vi "JKI.vi"() -> ()   [LabVIEW 2020]
uses:
  <userlib>/sushu/Tools/Front Panel State.ctl
  <vilib>/Utility/error.llb/Trim Whitespace.vi
  <userlib>/sushu/sushu.lvlib
panel:
  in  "OK":bool
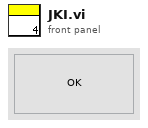
[diagram p1: front panel]
types:
  T1 = cluster{"Current VI Reference":refnum<vi>, "Close Panel on Exit?":bool}
  T2 = cluster{"Core":cluster{"Current VI Reference":refnum<vi>, "Close Panel on Exit?":bool}}
  T3 = enum32{"invalid app kind", "Development System", "Run Time System", "Student Edition", "Embedded LabVIEW", "Evaluation", "Custom"}
  T4 = typedef "sushu.lvlib/Front Panel State.ctl" = string
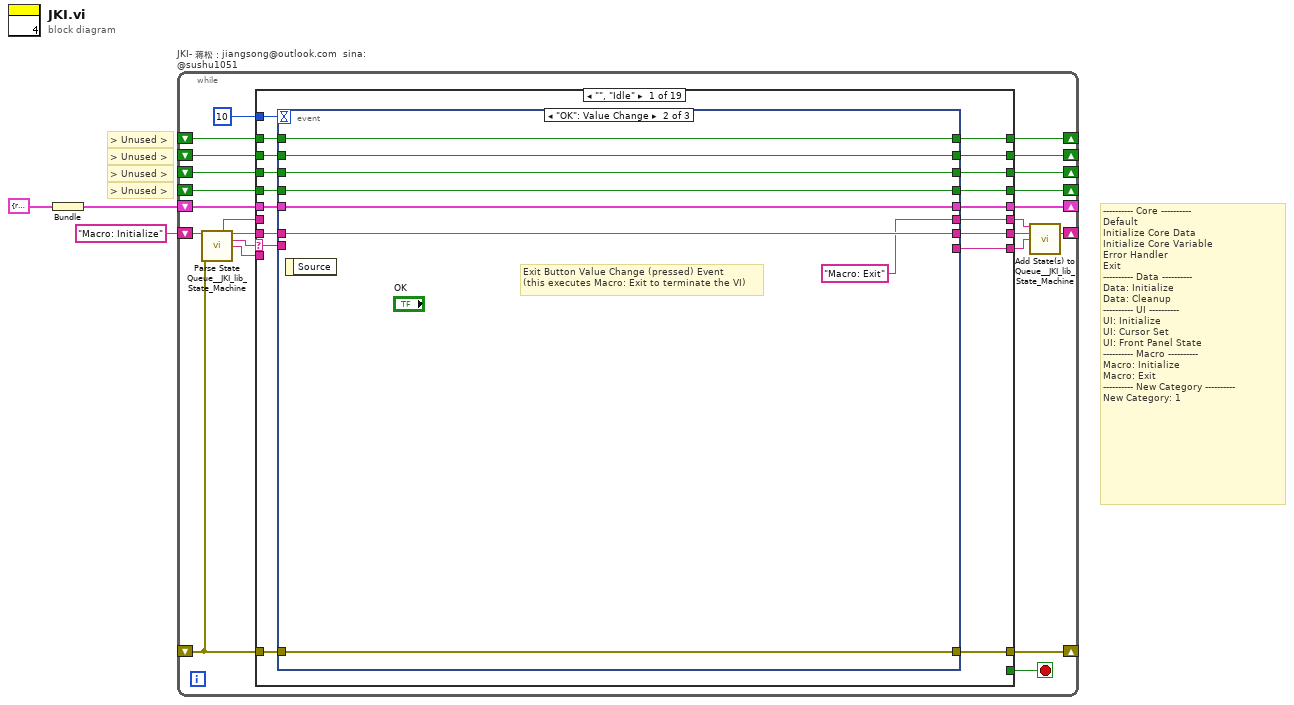
[diagram p0: block diagram]
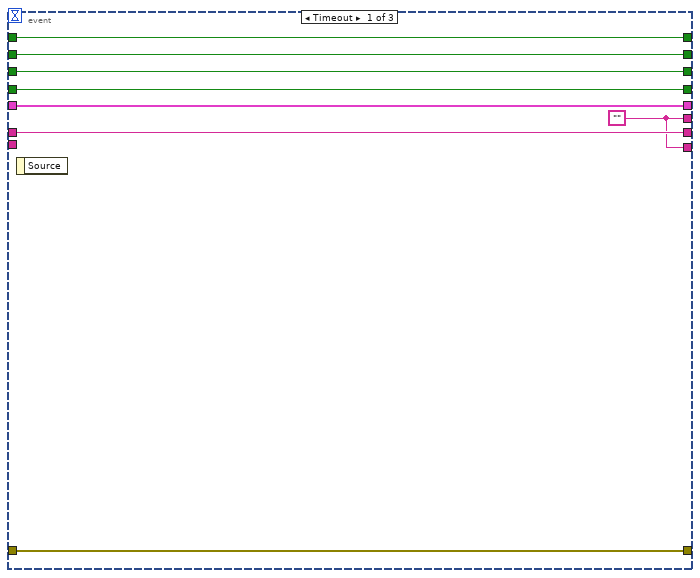
[diagram p2: hidden frame]
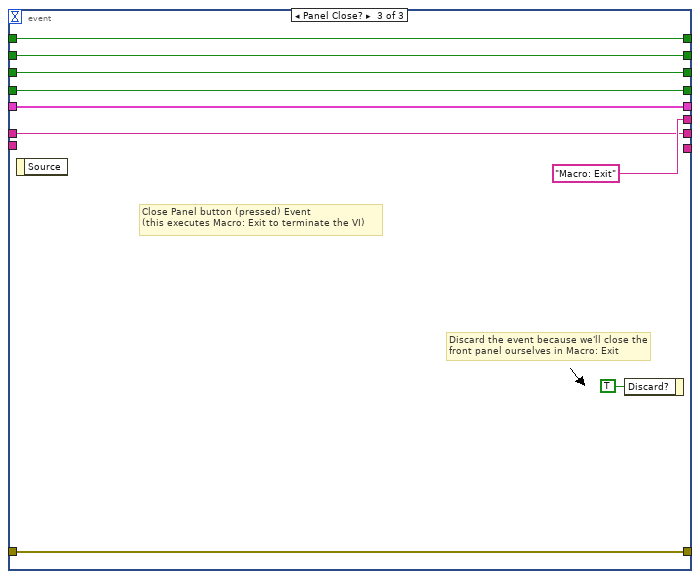
[diagram p3: hidden frame]
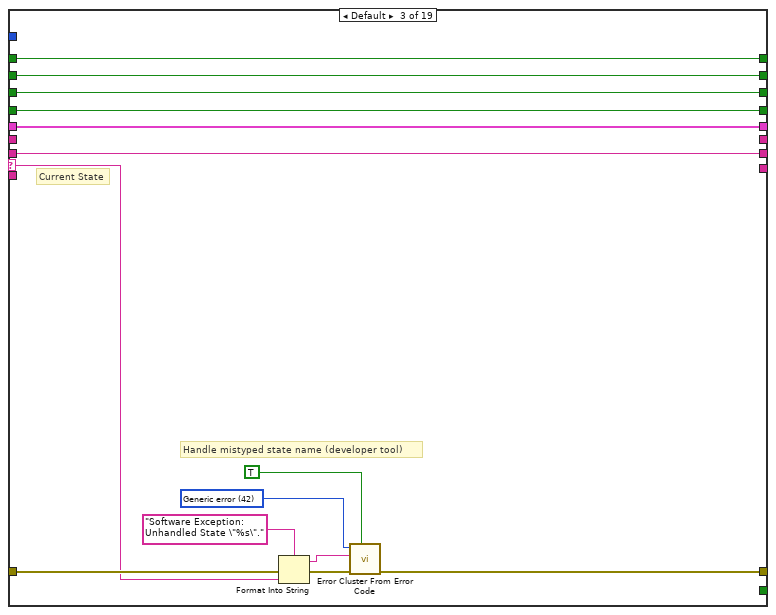
[diagram p5: hidden frame]
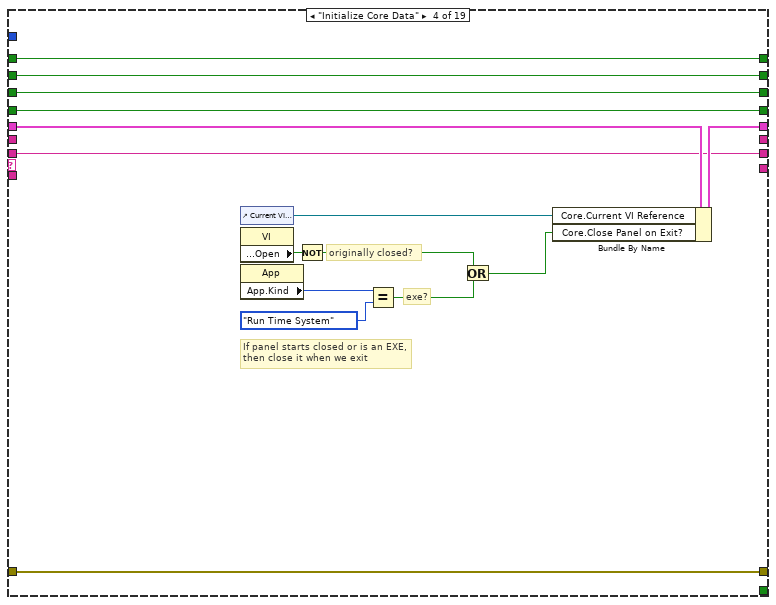
[diagram p6: hidden frame]
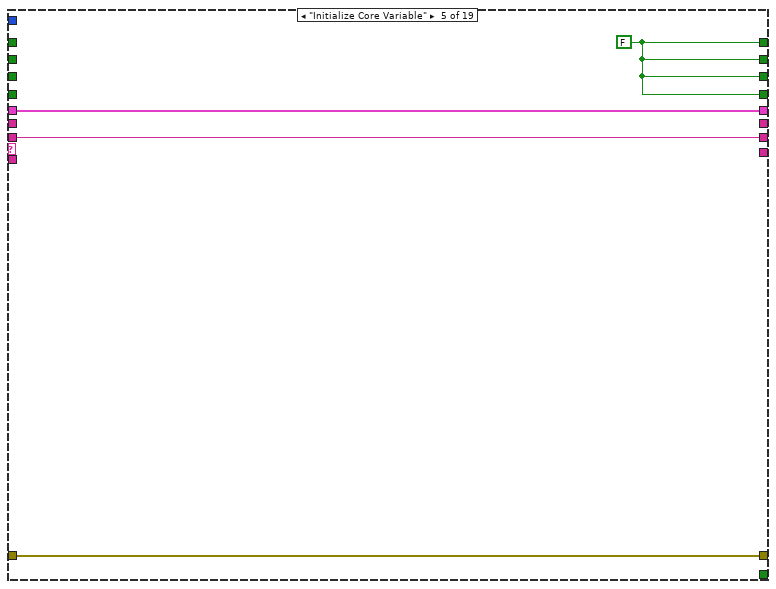
[diagram p7: hidden frame]
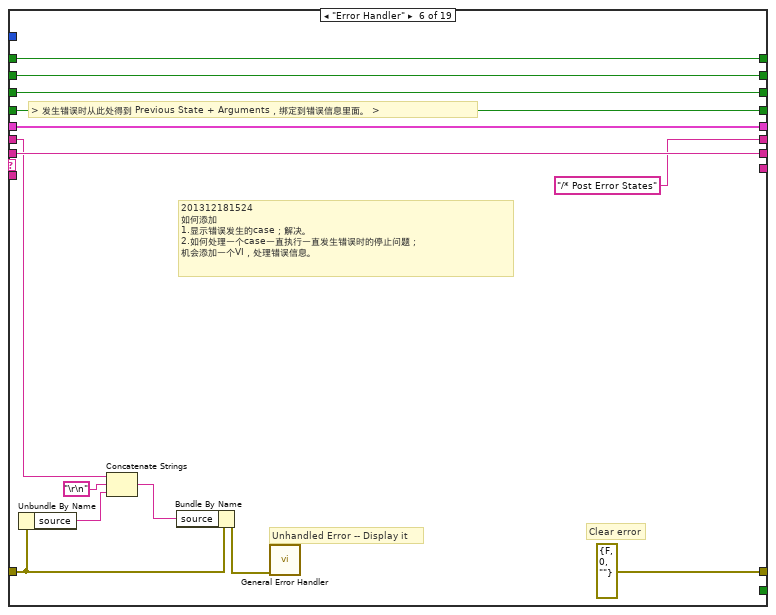
[diagram p8: hidden frame]
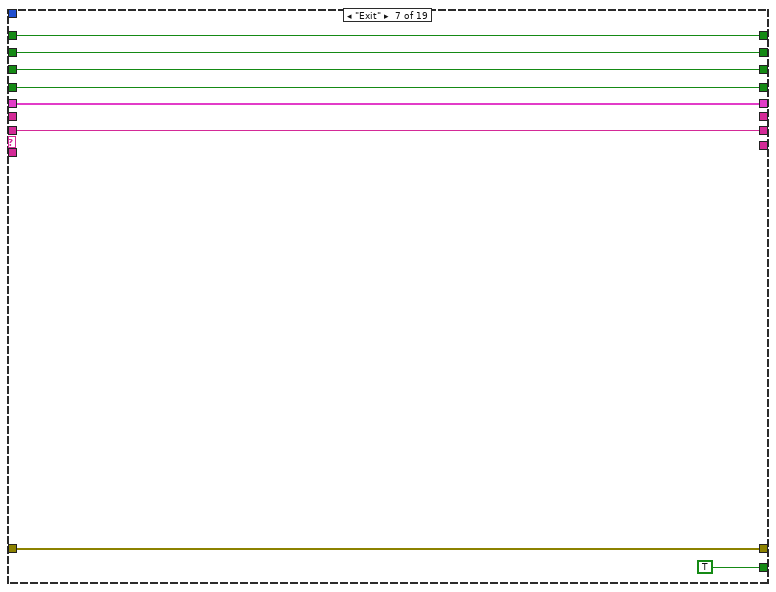
[diagram p9: hidden frame]
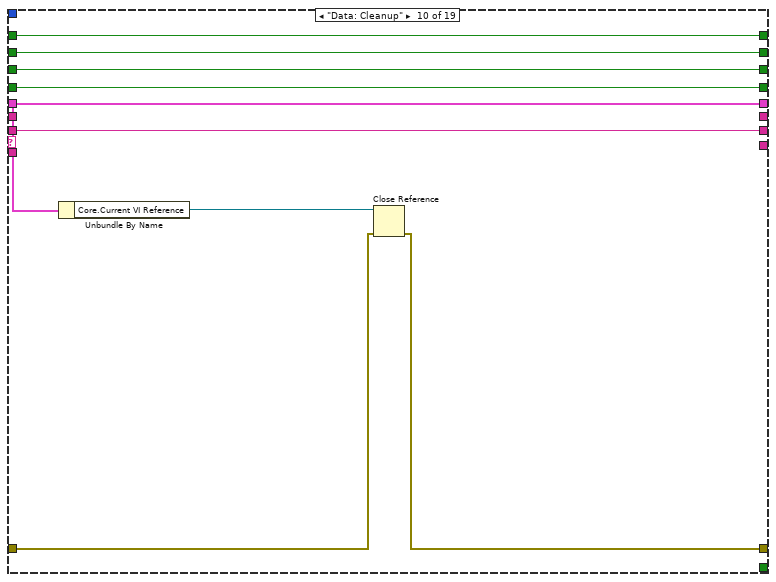
[diagram p12: hidden frame]
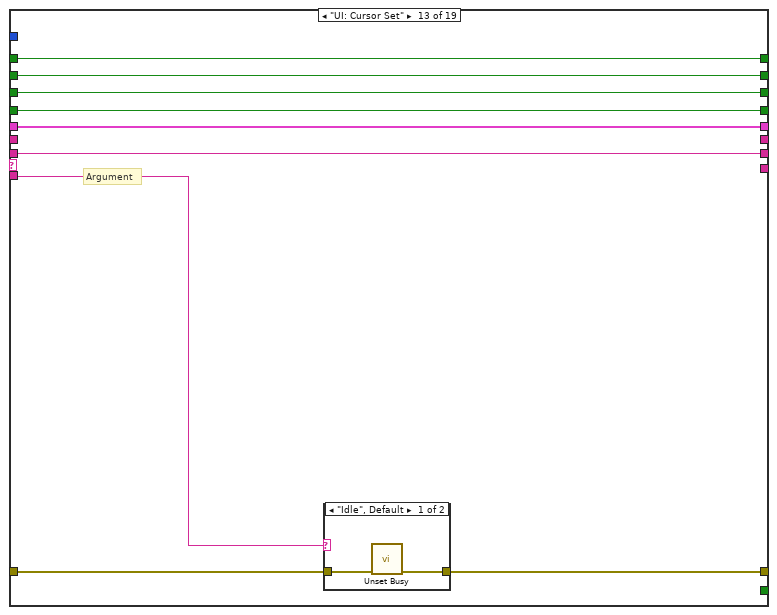
[diagram p15: hidden frame]
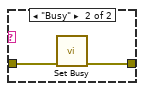
[diagram p16: hidden frame]
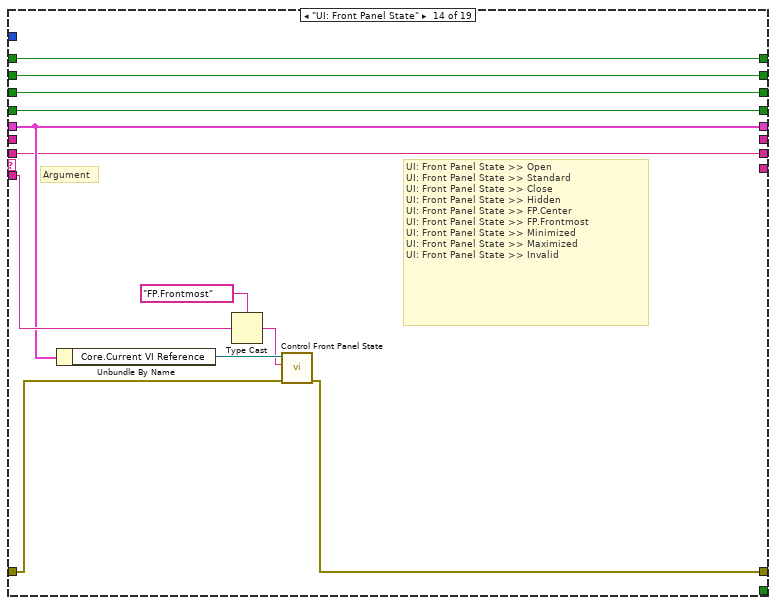
[diagram p17: hidden frame]
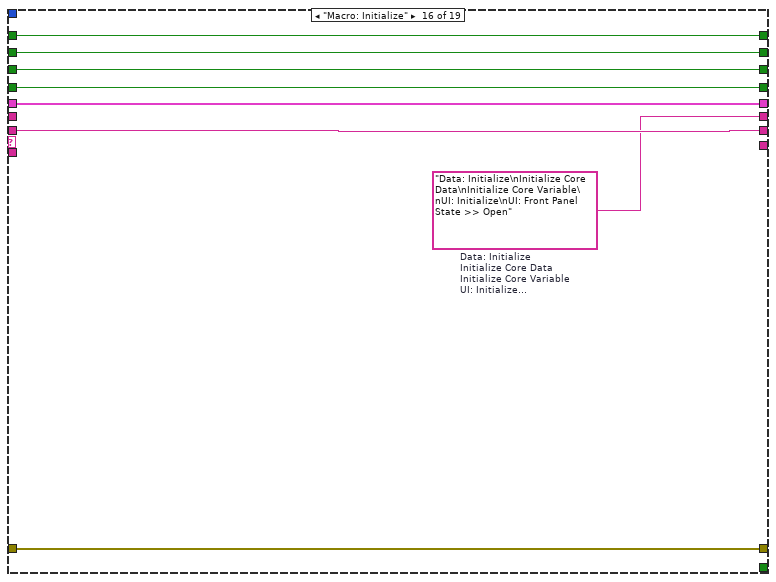
[diagram p19: hidden frame]
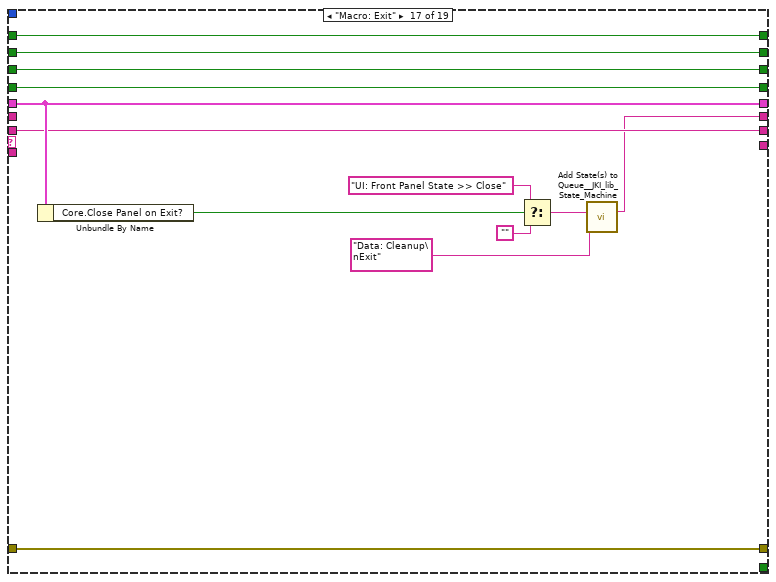
[diagram p20: hidden frame]
diagram:
  # "> Unused >"
  # "> Unused >"
  # "> Unused >"
  # "> Unused >"
  # "---------- Core ----------\nDefault\nInitialize Core Data\nInitialize Core Variable\nError Handler\nExit\n---------- Data ----------\nData: Initialize\nData: Cleanup\n---------- UI ----------\nUI: Initialize\nUI: Cursor Set\nUI: Front Panel State\n---------- Macro ----------\nMacro: Initialize\nMacro: Exit\n---------- New Category ----------\nNew Category: 1"
  n1 = Bundle("Core"=T1 {"Current VI Reference"=refnum, "Close Panel on Exit?"=FALSE}) -> (w1:T2)  [unwired: 1 in]
  n2 = while "JKI- 蒋松：jiangsong@outlook.com  sina: @sushu1051" {
    shift-right: [w23] -> _
    shift-left: _ -> [w20]
    shift-right: [w9] -> _
    shift-left: "Macro: Initialize" -> [w10]
    shift-right: [w16] -> _
    shift-left: _ -> [w18]
    shift-right: [w17] -> _
    shift-left: _ -> [w19]
    shift-right: [w11] -> _
    shift-left: w1 -> [w14]
    shift-right: [w12] -> _
    shift-left: _ -> [w5]
    shift-right: [w13] -> _
    shift-left: _ -> [w15]
    stop <- w22 stop-if-true
    n3 = call <vilib>:"Parse State Queue__JKI_lib_State_Machine.vi"("State Queue"=w10, "Error In (no error)"=w20) -> ("Previous State"=w4:string, "Remaining States"=w25:string, "Current State"=w26:string, "Arguments"=w24:string)  [unwired: 10 in]
    n4 = case shown="\"\", \"Idle\"" w26 {
      selector: w26 -> [w30 _ w78 _ _ _ _ _ _ _ _ _ _ _ _ _ _ _ _]
      tunnel: w25 -> [w44 w70 w77 w91 w107 w113 w124 w132 w140 w146 w155 w162 w169 w185 w194 w202 w210 w222 w229]
      tunnel: w24 -> [_ _ _ _ _ _ _ _ _ _ _ _ w173 w188 _ _ _ _ _]
      tunnel: [w42 w76 w79 w102 w109 errorcluster {"status"=FALSE, "code"=0, "source"=""} ("error out") w126 w134 w142 w148 w157 w164 w171 w189 w196 w204 w218 w225 w232] -> w23
      tunnel: w20 -> [w41 w76 w80 w102 w109 w117 w126 w134 w142 w149 w157 w164 w172 w190 w196 w204 w218 w225 w232]
      tunnel: [w43 w70 w77 w91 w107 w113 w124 w132 w140 w146 w155 w162 w169 w185 w194 w202 w210 w222 w229] -> w8
      tunnel: [_ _ _ _ _ _ TRUE _ _ _ _ _ _ _ _ _ _ _ _] -> w22
      tunnel: 10 ("Timeout") -> [w40 _ _ _ _ _ _ _ _ _ _ _ _ _ _ _ _ _ _]
      tunnel: w19 -> [w39 w75 w90 w105 _ w123 w131 w138 w145 w154 w161 w168 w177 w193 w200 w208 w221 w228 w235]
      tunnel: w18 -> [w38 w74 w89 w104 _ w122 w130 w137 w144 w153 w160 w167 w176 w192 w199 w207 w220 w227 w234]
      tunnel: [w37 w75 w90 w105 w106 w123 w131 w138 w145 w154 w161 w168 w177 w193 w200 w208 w221 w228 w235] -> w17
      tunnel: [w36 w74 w89 w104 w106 w122 w130 w137 w144 w153 w160 w167 w176 w192 w199 w207 w220 w227 w234] -> w16
      tunnel: w15 -> [w34 w73 w88 w103 _ w121 w129 w136 w143 w152 w159 w166 w175 w191 w198 w206 w219 w226 w233]
      tunnel: w5 -> [w33 w71 w87 w92 _ w111 w125 w133 w141 w147 w156 w163 w170 w186 w195 w203 w211 w223 w230]
      tunnel: w14 -> [w31 w72 w86 w94 w108 w120 w128 w135 w139 w150 w158 w165 w174 w187 w197 w205 w212 w224 w231]
      tunnel: [w35 w73 w88 w103 w106 w121 w129 w136 w143 w152 w159 w166 w175 w191 w198 w206 w219 w226 w233] -> w13
      tunnel: [w29 w71 w87 w92 w106 w111 w125 w133 w141 w147 w156 w163 w170 w186 w195 w203 w211 w223 w230] -> w12
      tunnel: [w32 w72 w86 w93 w108 w120 w128 w135 w139 w150 w158 w165 w174 w187 w197 w205 w212 w224 w231] -> w11
      tunnel: [w28 _ _ _ _ "/* Post Error States" _ _ _ _ _ _ _ _ _ w201 w209 _ _] -> w7
      tunnel: [w27 _ _ _ _ _ _ _ _ _ _ _ _ _ _ _ _ _ _] -> w6
      tunnel: w4 -> [_ _ _ _ _ w110 _ _ _ _ _ _ _ _ _ _ _ _ _]
      frame "", "Idle" {
        n5 = event shown="[1] \"OK\": Value Change" {
          selector: _ -> [_ _ _]
          dyn-events: _ -> [_ _ _]
          timeout: w40 -> [_ _ _]
          tunnel: w44 -> [w46 w54 w61]
          tunnel: [w46 w54 w61] -> w43
          tunnel: [w52 w60 w69] -> w42
          tunnel: w41 -> [w52 w60 w69]
          tunnel: w39 -> [w51 w59 w68]
          tunnel: w38 -> [w50 w58 w67]
          tunnel: [w51 w59 w68] -> w37
          tunnel: [w50 w58 w67] -> w36
          tunnel: [w49 w57 w66] -> w35
          tunnel: w34 -> [w49 w57 w66]
          tunnel: w33 -> [w47 w55 w63]
          tunnel: [w48 w56 w65] -> w32
          tunnel: w31 -> [w48 w56 w65]
          tunnel: w30 -> [_ _ _]
          tunnel: [w47 w55 w63] -> w29
          tunnel: [w45 "Macro: Exit" "Macro: Exit"] -> w28
          tunnel: [w45 _ _] -> w27
          event Timeout {
            w45 = ""
            n6 = event-data() -> ()  [unwired: 1 in, 1 out]
          }
          event "OK": Value Change {
            # "Exit Button Value Change (pressed) Event\n(this executes Macro: Exit to terminate the VI)"
            n7 = event-data() -> ()  [unwired: 1 in, 1 out]
          }
          event Panel Close? {
            # "Discard the event because we'll close the front panel ourselves in Macro: Exit"
            # "Close Panel button (pressed) Event\n(this executes Macro: Exit to terminate the VI)"
            n8 = event-data() -> ()  [unwired: 1 in, 1 out]
            n9 = event-data("Discard?"=TRUE) -> ()  [unwired: 1 in, 1 out]
          }
        }
      }
      frame "---------- Core ----------" {
      }
      frame Default {
        w82 = 42 items=["No error", "Argument error", "Memory is full", "Out of zone", "End of file", "File already open", "Generic file I/O error", "File not found", "File permission error", "Disk is full", "Duplicate path", "Too many files open", "System feature not enabled", "Resource file not found", "Cannot add resource", "Resource not found", "Image not found", "Image memory error", "Pen does not exist", "Config type invalid", "Config token not found", "Config parse error", "Config memory error", "Bad external code format", "Bad external code offset", "External code not present", "Null window", "Destroy window error", "Null menu", "Print aborted", "Bad print record", "Print driver error", "Windows error during printing", "Memory error during printing", "Print dialog error", "Generic print error", "Invalid device refnum", "Device not found", "Device parameter error", "Device unit error", "Cannot open device", "Device call aborted", "Generic error", "Cancelled by user", "Object ID too low", "Object ID too high", "Object not in heap", "Unknown heap", "Unknown object (invalid DefProc)", "Unknown object (DefProc not in table)", "Message out of range", "Invalid (null) method", "Unknown message", "Manager call not supported", "Bad address", "Network operation in progress", "Network operation timed out", "Connection is busy", "Network attribute not supported", "Network error", "Address in use", "System out of memory", "Connection aborted", "Connection refused", "Not connected", "Already connected", "Connection closed", "Initialization error (interapplication manager)", "Bad occurrence", "Wait on unbound occurrence handler", "Occurrence queue overflow", "Datalog type conflict", "Unused", "Unrecognized type (interapplication manager)", "Memory corrupt", "Failed to make temporary DLL", "Old CIN version", "Drag socket not found", "Failed to load drop-object", "Failed to register OLE object", "Failed to release OLE object", "Format specifier type mismatch", "Unknown format specifier", "Too few format specifiers", "Too many format specifiers", "Scan failed", "Newer CIN version", "Error converting to variant", "Runtime menu error", "Password tampered", "Variant attribute not found", "Incompatible variant data type", "Event data is not available", "Event Store is not present", "Occurrence is not found", "Event Queue is not created", "Event info is not available", "Refnum passed is NULL", "Error retrieving Class GUID", "Error retrieving CoClass GUID", "Error retrieving TypeLib GUID.", "Bad built application magic bytes.", "Specific driver is different from the specific driver associated with the Logical Name.", "There is no session opened to the class driver.", "Max Error", "MAX - Error with config objects", "MAX - Error loading configuration", "MAX - Group not supported"]
        # "Current State"
        # "Handle mistyped state name (developer tool)"
        n10 = Format Into String(format string="Software Exception: Unhandled State \"%s\"." ("message"), error in=w80, w78) -> (resulting string=w83:string, error out=w84:errorcluster)  [unwired: 1 in]
        n11 = call <vilib>:"Error Cluster From Error Code.vi"("show call chain? (False)"=TRUE, "error in (no error)"=w84, "error message (\"\")"=w83, "error code (0)"=w82) -> ("error out"=w79:errorcluster)  [unwired: 5 in]
      }
      frame "Initialize Core Data" {
        # "originally closed?"
        # "exe?"
        # "If panel starts closed or is an EXE, then close it when we exit"
        n12 = control-ref of="Current VI Reference"() -> (w101:refnum<vi>)
        n13 = property class="VI"() -> ("Front Panel.Open"=w95:bool)  [unwired: 2 in, 2 out]
        n14 = property class="App"() -> ("App.Kind"=w96:T3)  [unwired: 2 in, 2 out]
        n15 = Not(x=w95) -> (.not. x?=w98:bool)
        n16 = Equal?(x=w96, y=T3."Run Time System" ("Application:Kind")) -> (x = y?=w99:bool)
        n17 = Or(x=w98, y=w99) -> (x .or. y?=w100:bool)
        n18 = Bundle By Name(cluster=w94, "Core.Current VI Reference"=w101, "Core.Close Panel on Exit?"=w100) -> (w93:T2)
      }
      frame "Initialize Core Variable" {
        w106 = FALSE
      }
      frame "Error Handler" {
        # "> 发生错误时从此处得到 Previous State + Arguments，绑定到错误信息里面。 >"
        # "201312181524\n如何添加\n1.显示错误发生的case；解决。\n2.如何处理一个case一直执行一直发生错误时的停止问题；\n机会添加一个VI，处理错误信息。"
        # "Clear error"
        # "Unhandled Error -- Display it"
        n19 = Unbundle By Name(w117) -> ("source"=w115:string)
        n20 = Concatenate Strings(w110, "\r\n", w115) -> (w114:string)
        n21 = Bundle By Name(cluster=w117, "source"=w114) -> (w118:errorcluster)
        n22 = call <vilib>:"General Error Handler.vi"("error in (no error)"=w118) -> ()  [unwired: 10 in, 5 out]
      }
      frame "Exit" {
      }
      frame "---------- Data ----------" {
      }
      frame "Data: Initialize" {
      }
      frame "Data: Cleanup" {
        n23 = Unbundle By Name(w150) -> ("Core.Current VI Reference"=w151:refnum<vi>)
        n24 = Close Reference(reference=w151, error in (no error)=w149) -> (error out=w148:errorcluster)
      }
      frame "---------- UI ----------" {
      }
      frame "UI: Initialize" {
      }
      frame "UI: Cursor Set" {
        # "Argument"
        n25 = case shown="\"Idle\", Default" w173 {
          tunnel: w172 -> [w179 w181]
          tunnel: [w178 w180] -> w171
          frame "Idle", Default {
            n26 = call <vilib>:"Unset Busy.vi"("error in (no error)"=w179) -> ("error out"=w178:errorcluster)  [unwired: 10 in]
          }
          frame "Busy" {
            n27 = call <vilib>:"Set Busy.vi"("error in (no error)"=w181) -> ("error out"=w180:errorcluster)  [unwired: 9 in, 1 out]
          }
        }
      }
      frame "UI: Front Panel State" {
        # "UI: Front Panel State >> Open\nUI: Front Panel State >> Standard\nUI: Front Panel State >> Close\nUI: Front Panel State >> Hidden\nUI: Front Panel State >> FP.Center\nUI: Front Panel State >> FP.Frontmost\nUI: Front Panel State >> Minimized\nUI: Front Panel State >> Maximized\nUI: Front Panel State >> Invalid"
        # "Argument"
        n28 = Unbundle By Name(w187) -> ("Core.Current VI Reference"=w184:refnum<vi>)
        n29 = Type Cast(type=T4 "FP.Frontmost" ("Argument"), x=w188) -> (*(type *) &x=w183:T4)
        n30 = call <userlib>:"Control Front Panel State.vi"("error out"=w190, "Argument"=w183, "Core.Current VI Reference"=w184) -> ("error out"=w189:errorcluster)  [unwired: 7 in, 1 out]
      }
      frame "---------- Macro ----------" {
      }
      frame "Macro: Initialize" {
        w201 = "Data: Initialize\nInitialize Core Data\nInitialize Core Variable\nUI: Initialize\nUI: Front Panel State >> Open"  # Data: Initialize Initialize Core Data Initialize Core Variable UI: Initialize UI: Front Panel State >> Open
      }
      frame "Macro: Exit" {
        n31 = Unbundle By Name(w212) -> ("Core.Close Panel on Exit?"=w213:bool)
        n32 = Select(t="UI: Front Panel State >> Close", s=w213, f="") -> (s? t:f=w216:string)
        n33 = call <vilib>:"Add State(s) to Queue__JKI_lib_State_Machine.vi"("State(s) in (\"\")"=w216, "State(s) at Back (\"\")"="Data: Cleanup\nExit") -> ("States Out"=w209:string)  [unwired: 13 in]
      }
      frame "---------- New Category ----------" {
      }
      frame "New Category: 1" {
      }
    }
    n34 = call <vilib>:"Add State(s) to Queue__JKI_lib_State_Machine.vi"("State(s) in Front (\"\")"=w7, "State(s) in (\"\")"=w8, "State(s) at Back (\"\")"=w6) -> ("States Out"=w9:string)  [unwired: 12 in]
  }
